vi "gateway_main.vi"() -> ()   [LabVIEW 2012]
uses:
  <vilib>/Utility/miscctls.llb/LVRectTypeDef.ctl
panel:
  out "执行:状态":T1(ring)
  in  "停止":bool
  in  "节点":bool
  in  "历史":bool
  in  "主窗口":bool
  out "温度":cluster{sgl, sgl, sgl}(graph)
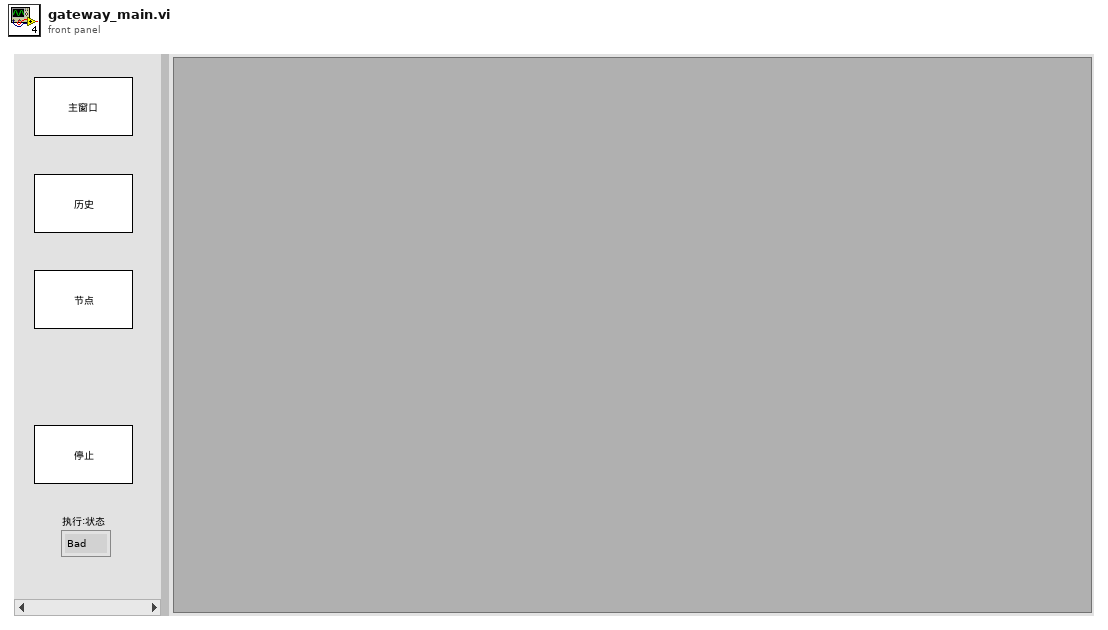
[diagram p1: front panel]
types:
  T1 = enum32{"Bad", "Idle", "Run top level", "Running"}
  T2 = cluster{"队列输出":refnum<queue>, "错误输出":errorcluster, "队列输出":refnum<queue>, "错误输出":errorcluster}
  T3 = typedef "LVRectTypeDef.ctl" = cluster{"Left":i16, "Top":i16, "Right":i16, "Bottom":i16}
  T4 = cluster{i32, enum16{"温度", "亮度", "电量", "连接质量"}, sgl}
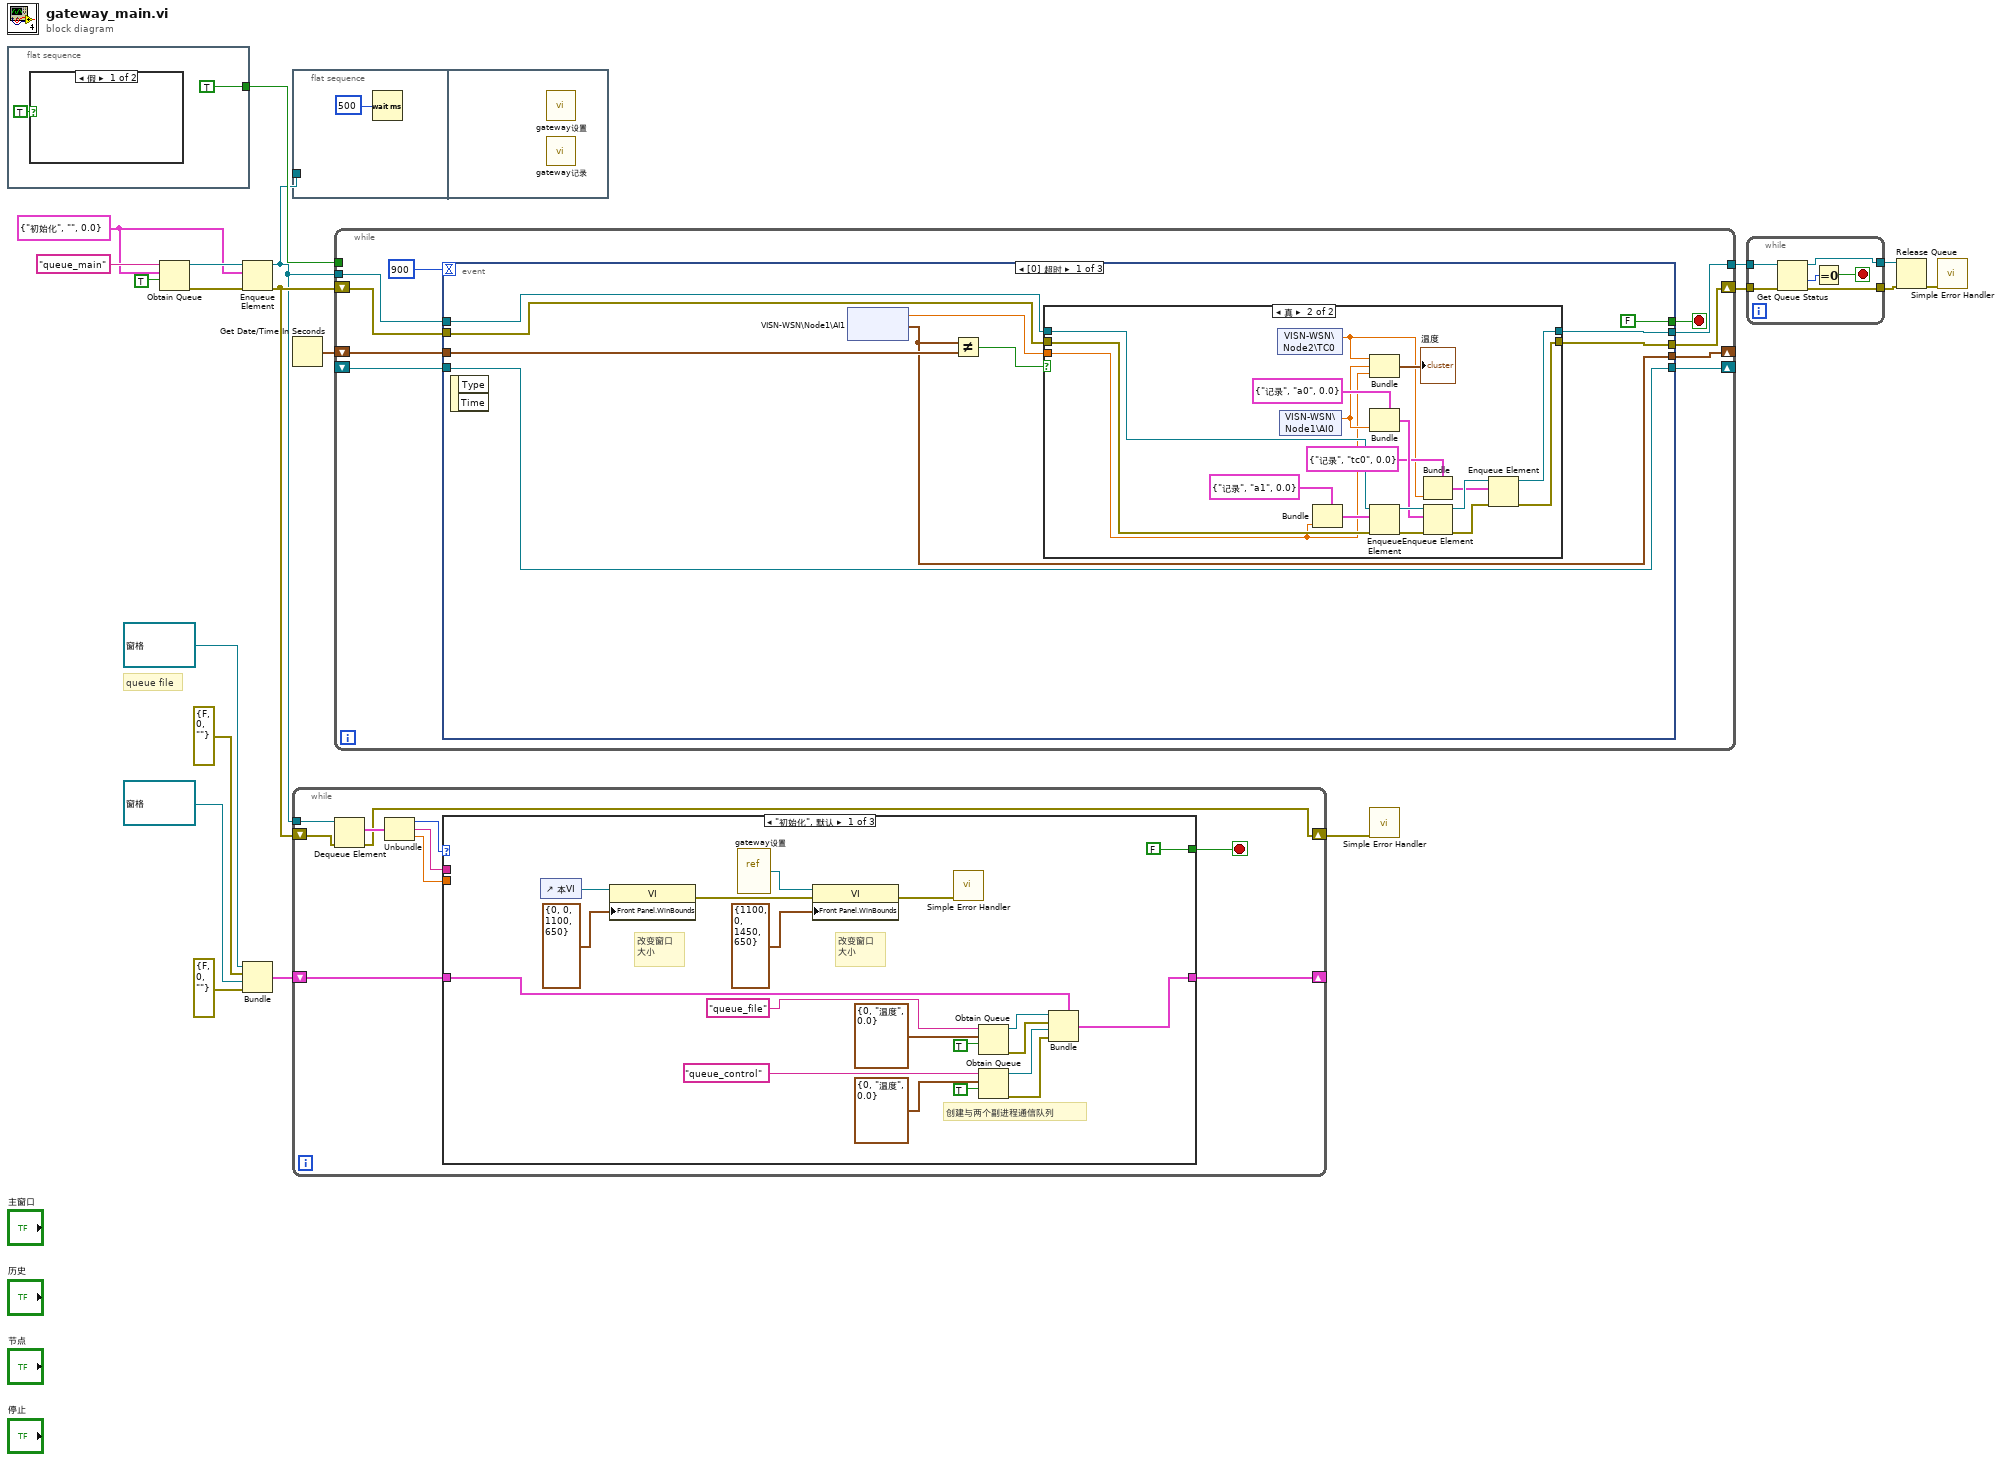
[diagram p0: block diagram]
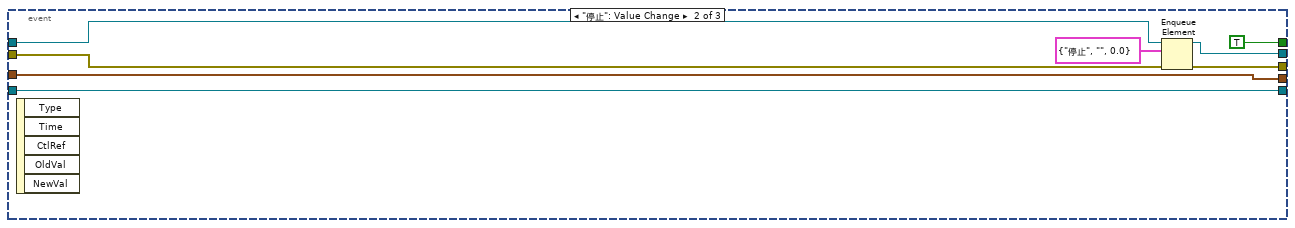
[diagram p3: hidden frame]
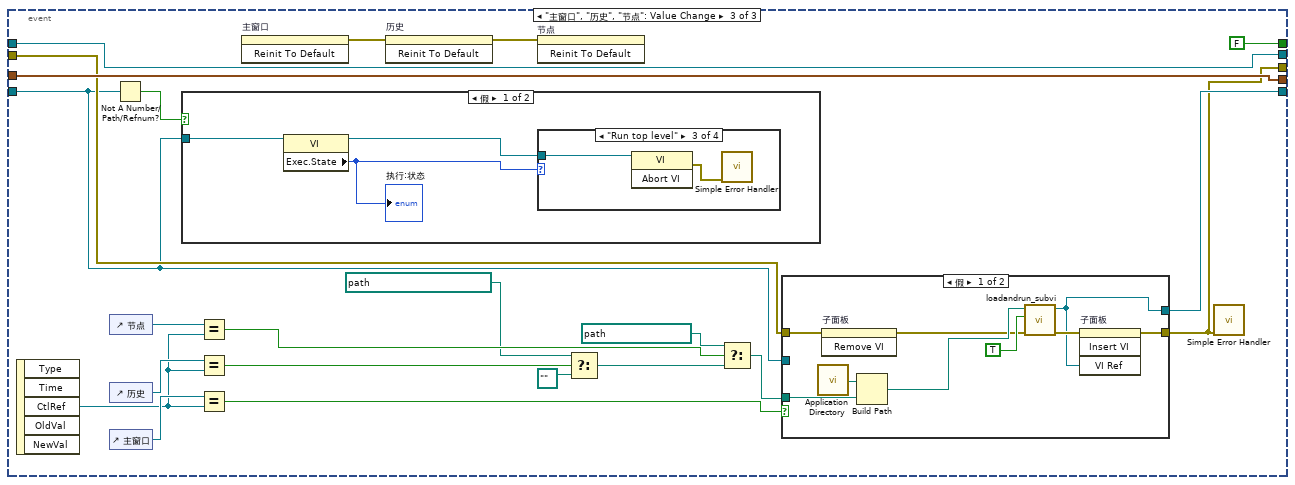
[diagram p4: hidden frame]
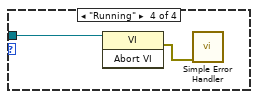
[diagram p7: hidden frame]
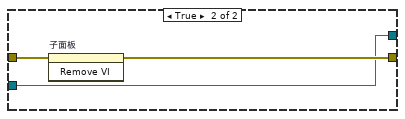
[diagram p9: hidden frame]
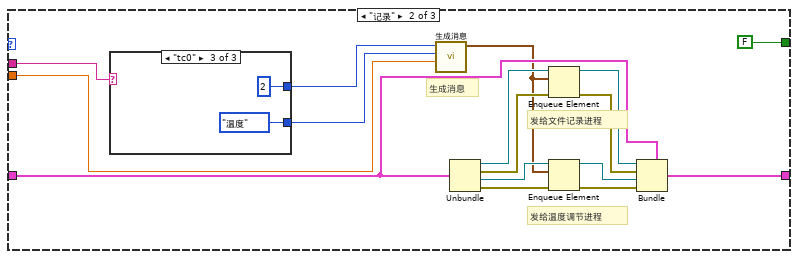
[diagram p10: hidden frame]
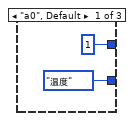
[diagram p11: hidden frame]
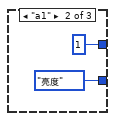
[diagram p12: hidden frame]
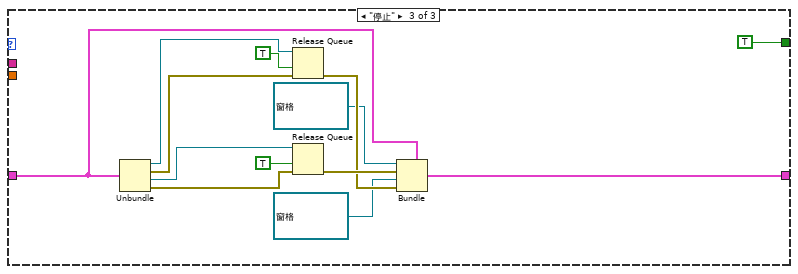
[diagram p13: hidden frame]
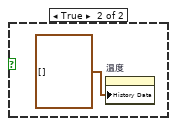
[diagram p14: hidden frame]
diagram:
  w11 = cluster{enum16{"初始化", "记录", "停止"}, string, dbl} {enum."初始化", "", 0.0}
  # "queue file"
  n1 = flat-sequence {
    tunnel: [TRUE] -> w4
    frame #0 {
      n2 = case shown="假" TRUE {
        frame False {
        }
        frame True {
          n3 = property on="温度" class="WFChart (严格)"("History Data"=cluster{sgl, sgl, sgl}[] [] ("历史数据")) -> ()  [unwired: 2 in, 2 out]
        }
      }
    }
  }
  n4 = Obtain Queue(name (unnamed)="queue_main" ("名称（未命名）"), element data type=w11, create if not found? (T)=TRUE ("如未找到是否创建？(T)")) -> (queue out=w16:refnum<queue>, error out=w15:errorcluster)  [unwired: 2 in, 1 out]
  n5 = Enqueue Element(queue=w16, element=w11, error in (no error)=w15) -> (queue out=w3:refnum<queue>, error out=w14:errorcluster)  [unwired: 1 in, 1 out]
  n6 = Bundle("队列输出"=refnum<queue> refnum, "错误输出"=errorcluster {"status"=FALSE, "code"=0, "source"=""}, "队列输出"=refnum<queue> refnum, "错误输出"=errorcluster {"status"=FALSE, "code"=0, "source"=""}) -> (w19:T2)  [unwired: 1 in]
  n7 = flat-sequence {
    tunnel: w3 -> [_]
    frame #0 {
      n8 = Wait (ms)(milliseconds to wait=u32 500 ("等待时间（毫秒）")) -> ()  [unwired: 1 out]
    }
    frame #1 {
      n9 = call "gateway设置.vi"() -> ()  [unwired: 12 in]
      n10 = call "gateway记录.vi"() -> ()  [unwired: 12 in]
    }
  }
  n11 = Get Date/Time In Seconds() -> (seconds since 1Jan1904=w13:timestamp)
  n12 = while {
    shift-right: [w32] -> _
    shift-left: w19 -> [w31]
    tunnel: w3 -> [w33]
    shift-right: [w25] -> w1
    shift-left: w14 -> [w34]
    stop <- w26 stop-if-true
    n13 = Dequeue Element(queue=w33, error in (no error)=w34) -> (element=w30:cluster{enum16{"初始化", "记录", "停止"}, string, dbl}, error out=w25:errorcluster)  [unwired: 1 in, 2 out]
    n14 = Unbundle(w30) -> (w29:enum16{"初始化", "记录", "停止"}, w28:string, w27:dbl)
    n15 = case shown="\"初始化\", 默认" w29 {
      tunnel: [w41 w64 w78] -> w32
      tunnel: w31 -> [w48 w65 w81]
      tunnel: w28 -> [_ w62 _]
      tunnel: w27 -> [_ w60 _]
      tunnel: [FALSE FALSE TRUE] -> w26
      frame "初始化", Default {
        # "改变窗口\n大小"
        # "改变窗口\n大小"
        # "创建与两个副进程通信队列"
        n16 = control-ref of="本VI"() -> (w40:refnum<vi>)
        n17 = property class="VI"(reference=w40, "Front Panel.WinBounds"=T3 {"Left"=0, "Top"=0, "Right"=1100, "Bottom"=650} ("前面板窗口:窗口边界")) -> (error out=w36:errorcluster)  [unwired: 1 in, 1 out]
        n18 = vi-ref "gateway设置.vi"() -> (w38:refnum<vi>)
        n19 = property class="VI"(reference=w38, error in=w36, "Front Panel.WinBounds"=T3 {"Left"=1100, "Top"=0, "Right"=1450, "Bottom"=650} ("前面板窗口:窗口边界")) -> (error out=w35:errorcluster)  [unwired: 1 out]
        n20 = call <vilib>:"Simple Error Handler.vi"("error in (no error)"=w35) -> ()  [unwired: 4 in, 5 out]
        n21 = Obtain Queue(name (unnamed)="queue_file" ("名称（未命名）"), element data type=T4 {0, enum."温度", 0.0}, create if not found? (T)=TRUE ("如未找到是否创建？(T)")) -> (queue out=w47:refnum<queue>, error out=w42:errorcluster)  [unwired: 2 in, 1 out]
        n22 = Obtain Queue(name (unnamed)="queue_control" ("名称（未命名）"), element data type=T4 {0, enum."温度", 0.0}, create if not found? (T)=TRUE ("如未找到是否创建？(T)")) -> (queue out=w44:refnum<queue>, error out=w43:errorcluster)  [unwired: 2 in, 1 out]
        n23 = Bundle(cluster=w48, "队列输出"=w47, "错误输出"=w42, "队列输出"=w44, "错误输出"=w43) -> (w41:T2)
      }
      frame "记录" {
        # "生成消息"
        # "发给文件记录进程"
        # "发给温度调节进程"
        n24 = case shown="\"tc0\"" w62 {
          tunnel: [1 ("节点ID") 1 ("节点ID") 2 ("节点ID")] -> w61
          tunnel: [enum16{"温度", "亮度", "电量", "连接质量"}."温度" ("属性") enum16{"温度", "亮度", "电量", "连接质量"}."亮度" ("属性") enum16{"温度", "亮度", "电量", "连接质量"}."温度" ("属性")] -> w59
          frame "a0", Default {
          }
          frame "a1" {
          }
          frame "tc0" {
          }
        }
        n25 = call "生成消息.vi"("值"=w60, "属性"=w59, "节点ID"=w61) -> ("输出簇"=w56:T4)  [unwired: 8 in]
        n26 = Unbundle(w65) -> ("队列输出"=w69:refnum<queue>, "错误输出"=w68:errorcluster, "队列输出"=w58:refnum<queue>, "错误输出"=w57:errorcluster)
        n27 = Enqueue Element(queue=w69, element=w56, error in (no error)=w68) -> (queue out=w67:refnum<queue>, error out=w66:errorcluster)  [unwired: 1 in, 1 out]
        n28 = Enqueue Element(queue=w58, element=w56, error in (no error)=w57) -> (queue out=w55:refnum<queue>, error out=w54:errorcluster)  [unwired: 1 in, 1 out]
        n29 = Bundle(cluster=w65, "队列输出"=w67, "错误输出"=w66, "队列输出"=w55, "错误输出"=w54) -> (w64:T2)
      }
      frame "停止" {
        n30 = Unbundle(w81) -> ("队列输出"=w87:refnum<queue>, "错误输出"=w86:errorcluster, "队列输出"=w84:refnum<queue>, "错误输出"=w83:errorcluster)
        n31 = Release Queue(queue=w87, force destroy? (F)=TRUE ("强制销毁？(F)"), error in (no error)=w86) -> (error out=w79:errorcluster)  [unwired: 2 out]
        n32 = Release Queue(queue=w84, force destroy? (F)=TRUE ("强制销毁？(F)"), error in (no error)=w83) -> (error out=w80:errorcluster)  [unwired: 2 out]
        n33 = Bundle(cluster=w81, "队列输出"=refnum<queue> refnum, "错误输出"=w80, "队列输出"=refnum<queue> refnum, "错误输出"=w79) -> (w78:T2)
      }
    }
  }
  n34 = while {
    tunnel: w3 -> [w98]
    shift-right: [w95] -> _
    shift-left: w13 -> [w96]
    tunnel: w4 -> [_]
    shift-right: [w92] -> w9
    shift-left: w14 -> [w91]
    tunnel: [w93] -> w10
    shift-right: [w90] -> _
    shift-left: _ -> [w89]
    stop <- w94 stop-if-true
    n35 = event shown="[0] 超时" {
      selector: _ -> [_ _ _]
      dyn-events: _ -> [_ _ _]
      timeout: 900 -> [_ _ _]
      tunnel: w98 -> [w105 w134 w144]
      tunnel: w96 -> [w108 w133 w145]
      tunnel: [w107 w133 w145] -> w95
      tunnel: [FALSE TRUE FALSE] -> w94
      tunnel: [w102 w135 w144] -> w93
      tunnel: [w100 w130 w137] -> w92
      tunnel: w91 -> [w101 w131 w141]
      tunnel: [w99 w129 w140] -> w90
      tunnel: w89 -> [w99 w129 w138]
      event Timeout {
        n36 = event-data() -> ()  [unwired: 1 in, 2 out]
        n37 = shared-variable "VISN-WSN\\Node1\\AI1"() -> (w104:sgl, w107:timestamp)  [unwired: 1 in, 1 out]
        n38 = Not Equal?(x=w107, y=w108) -> (x != y?=w106:bool)
        n39 = case shown="真" w106 {
          tunnel: w105 -> [w110 w128]
          tunnel: w104 -> [_ w111]
          tunnel: [w110 w119] -> w102
          tunnel: w101 -> [w109 w121]
          tunnel: [w109 w118] -> w100
          frame False {
          }
          frame True {
            n40 = shared-variable "VISN-WSN\\Node2\\TC0"() -> (w114:sgl)  [unwired: 1 in, 1 out]
            n41 = shared-variable "VISN-WSN\\Node1\\AI0"() -> (w112:sgl)  [unwired: 1 in, 1 out]
            n42 = Bundle(cluster=cluster{enum16{"初始化", "记录", "停止"}, string, dbl} {enum."记录", "a1", 0.0}, w111) -> (w126:cluster{enum16{"初始化", "记录", "停止"}, string, dbl})  [unwired: 2 in]
            n43 = Bundle(w114, w112, w111) -> (→"温度":cluster{sgl, sgl, sgl})  [unwired: 1 in]
            n44 = Bundle(cluster=cluster{enum16{"初始化", "记录", "停止"}, string, dbl} {enum."记录", "a0", 0.0}, w112) -> (w123:cluster{enum16{"初始化", "记录", "停止"}, string, dbl})  [unwired: 2 in]
            n45 = Enqueue Element(queue=w128, element=w126, error in (no error)=w121) -> (queue out=w125:refnum<queue>, error out=w122:errorcluster)  [unwired: 1 in, 1 out]
            n46 = Bundle(cluster=cluster{enum16{"初始化", "记录", "停止"}, string, dbl} {enum."记录", "tc0", 0.0}, w114) -> (w113:cluster{enum16{"初始化", "记录", "停止"}, string, dbl})  [unwired: 2 in]
            n47 = Enqueue Element(queue=w125, element=w123, error in (no error)=w122) -> (queue out=w116:refnum<queue>, error out=w117:errorcluster)  [unwired: 1 in, 1 out]
            n48 = Enqueue Element(queue=w116, element=w113, error in (no error)=w117) -> (queue out=w119:refnum<queue>, error out=w118:errorcluster)  [unwired: 1 in, 1 out]
          }
        }
      }
      event "停止": Value Change {
        n49 = event-data() -> ()  [unwired: 1 in, 5 out]
        n50 = Enqueue Element(queue=w134, element=cluster{enum16{"初始化", "记录", "停止"}, string, dbl} {enum."停止", "", 0.0}, error in (no error)=w131) -> (queue out=w135:refnum<queue>, error out=w130:errorcluster)  [unwired: 1 in, 1 out]
      }
      event "主窗口", "历史", "节点": Value Change {
        n51 = event-data() -> ("CtlRef"=w156:refnum<vi>)  [unwired: 1 in, 4 out]
        n52 = control-ref of="节点"() -> (w155:refnum<vi>)
        n53 = control-ref of="历史"() -> (w158:refnum<vi>)
        n54 = control-ref of="主窗口"() -> (w157:refnum<vi>)
        n55 = Not A Number/Path/Refnum?(number/path/refnum=w138) -> (NaN/Path/Refnum?=w139:bool)
        n56 = case shown="假" w139 {
          tunnel: w138 -> [w161 _]
          frame False {
            n57 = property class="VI"(reference=w161) -> (reference out=w159:refnum<vi>, "Exec.State"=w160:T1)  [unwired: 1 in, 1 out]
            "执行:状态" <- w160
            n58 = case shown="\"Run top level\"" w160 {
              tunnel: w159 -> [_ _ w162 w165]
              frame "Bad", Default {
              }
              frame "Idle" {
              }
              frame "Run top level" {
                n59 = invoke class="VI" method="Abort VI"(reference=w162) -> (error out=w163:errorcluster)  [unwired: 2 in, 2 out]
                n60 = call <vilib>:"Simple Error Handler.vi"("error in (no error)"=w163) -> ()  [unwired: 4 in, 5 out]
              }
              frame "Running" {
                n61 = invoke class="VI" method="Abort VI"(reference=w165) -> (error out=w164:errorcluster)  [unwired: 2 in, 2 out]
                n62 = call <vilib>:"Simple Error Handler.vi"("error in (no error)"=w164) -> ()  [unwired: 4 in, 5 out]
              }
            }
          }
          frame True {
          }
        }
        n63 = Equal?(x=w155, y=w156) -> (x = y?=w154:bool)
        n64 = Equal?(x=w158, y=w156) -> (x = y?=w153:bool)
        n65 = Equal?(x=w157, y=w156) -> (x = y?=w148:bool)
        n66 = invoke on="主窗口" class="Bool" method="Reinit To Default"() -> (error out=w143:errorcluster)  [unwired: 3 in, 2 out]
        n67 = invoke on="历史" class="Bool" method="Reinit To Default"(error in=w143) -> (error out=w142:errorcluster)  [unwired: 2 in, 2 out]
        n68 = invoke on="节点" class="Bool" method="Reinit To Default"(error in=w142) -> ()  [unwired: 2 in, 3 out]
        n69 = Select(t=path "gateway打开历史文件.vi", s=w153, f=path "") -> (s? t:f=w150:path)
        n70 = Select(t=path "gateway发消息.vi", s=w154, f=w150) -> (s? t:f=w147:path)
        n71 = case shown="假" w148 {
          tunnel: w147 -> [w173 _]
          tunnel: [w169 w177] -> w137
          tunnel: w141 -> [w168 w176]
          tunnel: [w166 w175] -> w140
          tunnel: w138 -> [_ w175]
          frame False {
            n72 = call <vilib>:"Application Directory.vi"() -> ("Application Directory"=w174:path)
            n73 = invoke on="子面板" class="SubPnl" method="Remove VI"(error in=w168) -> (error out=w167:errorcluster)  [unwired: 2 in, 2 out]
            n74 = Build Path(base path=w174, name or relative path=w173) -> (appended path=w172:path)
            n75 = call "loadandrun_subvi.vi"("path"=w172, "run?"=TRUE, "error in (no error)"=w167) -> ("vi refnum out"=w166:refnum<vi>, "error out"=w170:errorcluster)  [unwired: 6 in]
            n76 = invoke on="子面板" class="子面板" method="Insert VI"(error in=w170, "VI Ref"=w166) -> (error out=w169:errorcluster)  [unwired: 2 in, 3 out]
          }
          frame True {
            n77 = invoke on="子面板" class="SubPnl" method="Remove VI"(error in=w176) -> (error out=w177:errorcluster)  [unwired: 2 in, 2 out]
          }
        }
        n78 = call <vilib>:"Simple Error Handler.vi"("error in (no error)"=w137) -> ()  [unwired: 4 in, 5 out]
      }
    }
  }
  n79 = call <vilib>:"Simple Error Handler.vi"("error in (no error)"=w1) -> ()  [unwired: 4 in, 5 out]
  n80 = while {
    tunnel: w10 -> [w183]
    tunnel: w9 -> [w182]
    tunnel: [w179] -> w8
    tunnel: [w178] -> w7
    stop <- w180 stop-if-true
    n81 = Get Queue Status(queue=w183, error in (no error)=w182) -> (queue out=w179:refnum<queue>, # pending insert=w181:i32, error out=w178:errorcluster)  [unwired: 1 in, 5 out]
    n82 = Equal To 0?(x=w181) -> (x = 0?=w180:bool)
  }
  n83 = Release Queue(queue=w8, error in (no error)=w7) -> (error out=w2:errorcluster)  [unwired: 1 in, 2 out]
  n84 = call <vilib>:"Simple Error Handler.vi"("error in (no error)"=w2) -> ()  [unwired: 4 in, 5 out]
